vi "niScope EX Advanced Measurement Library.vi"() -> ()   [LabVIEW 2021]
doc: "Example: Advanced Measurement Library\n\nRecommended Input Signal: 100 kHz, 1 Vpp, sine wave\n\nDevices Supported: Refer to NI Example Finder\n\nLabVIEW Description:\n\nThis example illustrates using some of the advanced measurement library functions such as waveform processing. The example calls Auto Setup once to configure the vertical and horizontal subsystems of the digitizer based on the input to all the channels. \n\nThe property node is used to set some of the common filter parameters. For more information about measurement library parameters, see the NI-SCOPE VI Reference help file. The NI High Speed Digitizers Help also offers an introduction to the analysis algorithms provided in NI-SCOPE. \n\nWhen Add Waveform Processing VI is called, all the waveform measurement parameters are cached. Before any measurements are retrieved, that set of parameters is used to perform the processing measurement on the acquired waveform.\n\nIn this example, both the call to Fetch Measurement and Fetch Array Measurement are computed using the result of the processing step. Use the \"None\" array measurement function to retrieve only the processed waveform.\n\nThe Clear Waveform Processing VI is called during each loop iteration. This is necessary since we add a processing step every loop so you can change the processing measurement while the VI is executing. Alternatively, if the processing measurement never changes we could add one processing step outside the loop and never clear it."
uses:
  <instrlib>/niScope/Acquire/niScope Multi Read Cluster.vi
  <instrlib>/niScope/Measurements/niScope Fetch Measurement.vi
  <instrlib>/niScope/Measurements/niScope Multi Fetch Array Measurement Cluster.vi
panel:
  in  "Array Measurement":i32(ring)=4019 items=["None"=4000, "Last Acq. Histogram"=4001, "Multi Acq. Voltage Histogram"=4004, "Multi Acq. Time Histogram"=4005, "Multi Acq. Average"=4016, "Polynomial Interpolation"=4011, "Array Integral"=4006, "Derivative"=4007, "Inverse"=4008, "Multiply Channels"=4012, "Add Channels"=4013, "Subtract Channels"=4014, "Divide Channels"=4015, "Array Offset"=4025, "Array Gain"=4026, "Hanning Window"=4009, "Flat Top Window"=4010, "Hamming Window"=4020, "Triangle Window"=4023, "Blackman Window"=4024, "FIR Windowed Filter"=4021, "Bessel IIR Filter"=4022, "Butterworth IIR Filter"=4017, "Chebyshev IIR Filter"=4018, "FFT Phase Spectrum"=4002, "FFT Amp. Spectrum (Volts RMS)"=4003, "FFT Amp. Spectrum (dB)"=4019]
  in  "Scalar Measurement":i32(ring)=1008 items=["None"=4000, "Frequency"=2, "Average Frequency"=1016, "FFT Frequency"=1008, "Period"=3, "Average Period"=1015, "Rise Time"=0, "Fall Time"=1, "Rising Slew Rate"=1010, "Falling Slew Rate"=1011, "Overshoot"=18, "Preshoot"=19, "Voltage RMS"=4, "Voltage Cycle RMS"=16, "AC Estimate"=1012, "FFT Amplitude"=1009, "Voltage Average"=10, "Voltage Cycle Average"=17, "DC Estimate"=1013, "Voltage Max"=6, "Voltage Min"=7, "Voltage Peak-to-Peak"=5, "Voltage High"=8, "Voltage Low"=9, "Voltage Amplitude"=15, "Voltage Top"=1007, "Voltage Base"=1006, "Voltage Base-to-Top"=1017, "Negative Width"=11, "Positive Width"=12, "Negative Duty Cycle"=13, "Positive Duty Cycle"=14, "Integral"=1005, "Area"=1003, "Cycle Area"=1004, "Time Delay"=1014, "Phase Delay"=1018, "Low Ref Volts"=1000, "Mid Ref Volts"=1001, "High Ref Volts"=1002, "Volt. Hist. Mean"=2000, "Volt. Hist. Stdev"=2001, "Volt. Hist. Median"=2003, "Volt. Hist. Mode"=2010, "Volt. Hist. Max"=2005, "Volt. Hist. Min"=2006, "Volt. Hist. Peak-to-Peak"=2002, "Volt. Hist. Mean + Stdev"=2007, "Volt. Hist. Mean + 2 Stdev"=2008, "Volt. Hist. Mean + 3 Stdev"=2009, "Volt. Hist. Hits"=2004, "Volt. Hist. New Hits"=2011, "Time Hist. Mean"=3000, "Time Hist. Stdev"=3001, "Time Hist. Median"=3003, "Time Hist. Mode"=3010, "Time Hist. Max"=3005, "Time Hist. Min"=3006, "Time Hist. Peak-to-Peak"=3002, "Time Hist. Mean + Stdev"=3007, "Time Hist. Mean + 2 Stdev"=3008, "Time Hist. Mean + 3 Stdev"=3009, "Time Hist. Hits"=3004, "Time Hist. New Hits"=3011]
  in  "Processing Step Measurement":i32(ring)=4000 items=["None"=4000, "Last Acq. Histogram"=4001, "Multi Acq. Voltage Histogram"=4004, "Multi Acq. Time Histogram"=4005, "Multi Acq. Average"=4016, "Polynomial Interpolation"=4011, "Array Integral"=4006, "Derivative"=4007, "Inverse"=4008, "Multiply Channels"=4012, "Add Channels"=4013, "Subtract Channels"=4014, "Divide Channels"=4015, "Array Offset"=4025, "Array Gain"=4026, "Hanning Window"=4009, "Flat Top Window"=4010, "Hamming Window"=4020, "Triangle Window"=4023, "Blackman Window"=4024, "FIR Windowed Filter"=4021, "Bessel IIR Filter"=4022, "Butterworth IIR Filter"=4017, "Chebyshev IIR Filter"=4018, "FFT Phase Spectrum"=4002, "FFT Amp. Spectrum (Volts RMS)"=4003, "FFT Amp. Spectrum (dB)"=4019]
  in  "Stop Button":bool
  out "Scalar Result":dbl
  out "Waveform Chart":T1(graph)
  out "Array Measurement Chart":T1(graph)
  in  "Channel(s)":string="0"
  in  "Resource Name":refnum<k15>="PXI1Slot2" caption="Resource Name(s)"
  in  "Bandpass/Stop Center Frequency (Hz)":dbl=100000.0 format="%#_6p"
  in  "Bandpass / Bandstop Width":dbl=1000.0 format="%#_6p"
  in  "Filter Type":i32(ring) items=["lowpass", "highpass", "bandpass", "bandstop"]
  in  "Low/Highpass Cutoff Frequency (Hz)":dbl=500000.0 format="%#_6p"
  # "Waveform Measurement Settings"
  # "Filter Parameters"
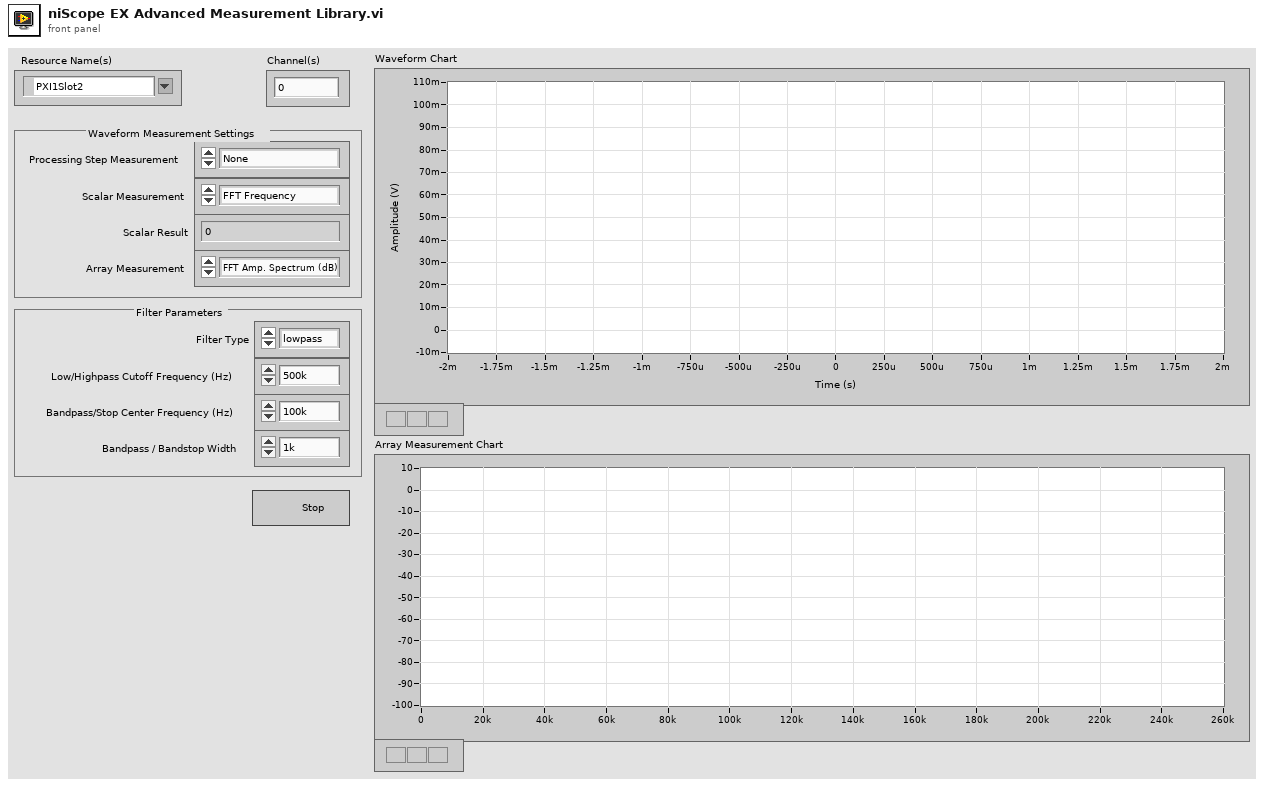
[diagram p1: front panel]
types:
  T1 = cluster{"relativeInitialX":dbl, "xIncrement":dbl, "measWfm":dbl[]}[]
  T2 = cluster{"relativeInitialX":dbl, "xIncrement":dbl, "wfm":dbl[]}[]
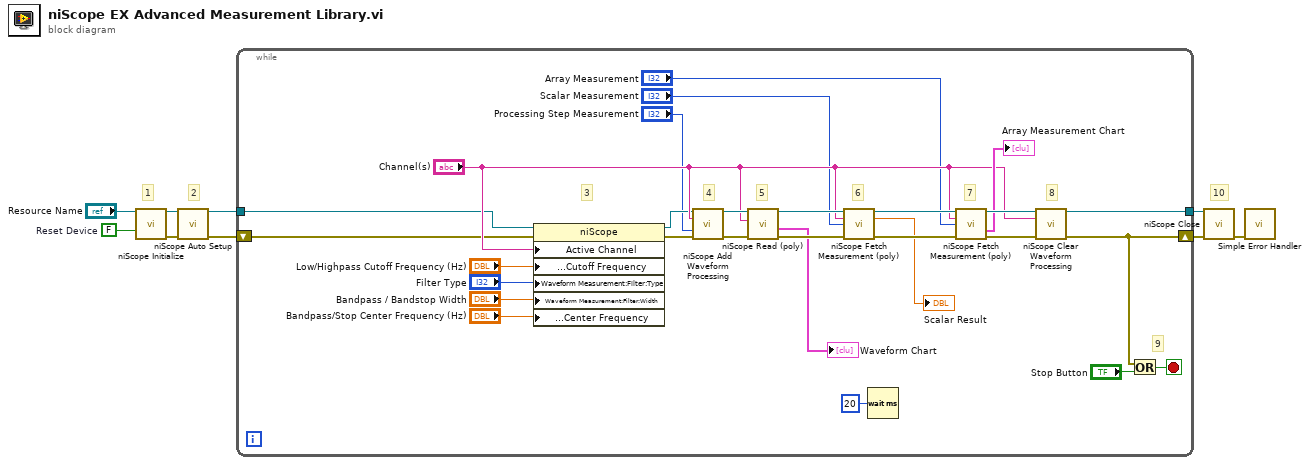
[diagram p0: block diagram]
diagram:
  w6 = FALSE  # Reset Device
  # "10"
  # "2"
  # "1"
  n1 = call <instrlib>:"niScope Initialize.vi"("resource name"="Resource Name", "reset device"=w6) -> ("instrument handle"=w9:refnum<k15>, "error out"=w8:errorcluster)  [unwired: 12 in]
  n2 = call <instrlib>:"niScope Auto Setup.vi"("instrument handle"=w9, "error in"=w8) -> ("instrument handle out"=w4:refnum<k15>, "error out"=w3:errorcluster)  [unwired: 12 in]
  n3 = while {
    tunnel: w4 -> [w13]
    tunnel: [w11] -> w2
    shift-right: [w10] -> w1
    shift-left: w3 -> [w12]
    stop <- w22 stop-if-true
    # "9"
    # "8"
    # "7"
    # "6"
    # "3"
    # "4"
    # "5"
    n4 = property class="niScope"(reference=w13, error in=w12, "Active Channel"="Channel(s)", "Waveform Measurement:Filter:Cutoff Frequency"="Low/Highpass Cutoff Frequency (Hz)", "Waveform Measurement:Filter:Type"="Filter Type", "Waveform Measurement:Filter:Width"="Bandpass / Bandstop Width", "Waveform Measurement:Filter:Center Frequency"="Bandpass/Stop Center Frequency (Hz)") -> (reference out=w17:refnum<k15>, error out=w37:errorcluster)
    n5 = call <instrlib>:"niScope Add Waveform Processing.vi"("instrument handle"=w17, "channels"="Channel(s)", "array measurement"="Processing Step Measurement", "error in"=w37) -> ("instrument handle out"=w32:refnum<k15>, "error out"=w31:errorcluster)  [unwired: 10 in]
    n6 = call-poly <instrlib>:"niScope Read (poly).vi"("error in"=w31, "channels"="Channel(s)", "instrument handle"=w32) -> ("error out"=w29:errorcluster, "waveform"=→"Waveform Chart":T2, "instrument handle out"=w30:refnum<k15>)  [unwired: 5 in, 1 out]
    n7 = call-poly <instrlib>:"niScope Fetch Measurement (poly).vi"("instrument handle"=w30, "channels"="Channel(s)", "scalar measurement"="Scalar Measurement", "error in"=w29) -> ("instrument handle out"=w28:refnum<k15>, "result"=→"Scalar Result":dbl, "error out"=w27:errorcluster)  [unwired: 9 in]
    n8 = Wait (ms)(milliseconds to wait=u32 20 ("millisecond multiple")) -> ()  [unwired: 1 out]
    n9 = call-poly <instrlib>:"niScope Fetch Measurement (poly).vi"("instrument handle"=w28, "channels"="Channel(s)", "array measurement"="Array Measurement", "error in"=w27) -> ("instrument handle out"=w26:refnum<k15>, "meas waveform"=→"Array Measurement Chart":T1, "error out"=w19:errorcluster)  [unwired: 8 in, 1 out]
    n10 = call <instrlib>:"niScope Clear Waveform Processing.vi"("instrument handle"=w26, "channels"="Channel(s)", "error in"=w19) -> ("instrument handle out"=w11:refnum<k15>, "error out"=w10:errorcluster)  [unwired: 11 in]
    n11 = Or(x=w10, y="Stop Button") -> (x .or. y?=w22:bool)
  }
  n12 = call <instrlib>:"niScope Close.vi"("instrument handle"=w2, "error in"=w1) -> ("error out"=w5:errorcluster)  [unwired: 13 in]
  n13 = call <vilib>:"Simple Error Handler.vi"("error in (no error)"=w5) -> ()  [unwired: 4 in, 5 out]
